vi "Run_Core.vi"(0 "Message Popup in":refnum<class "Wait.lvclass">, 11 "error in (no error)":errorcluster) -> (4 "Message Popup out":refnum<class "Wait.lvclass">, 6 "Return":variant, 15 "error out":errorcluster)   [LabVIEW 2016, in "Wait.lvclass"]
uses:
  Wait.lvclass
  Wait.lvclass/Wait.ctl
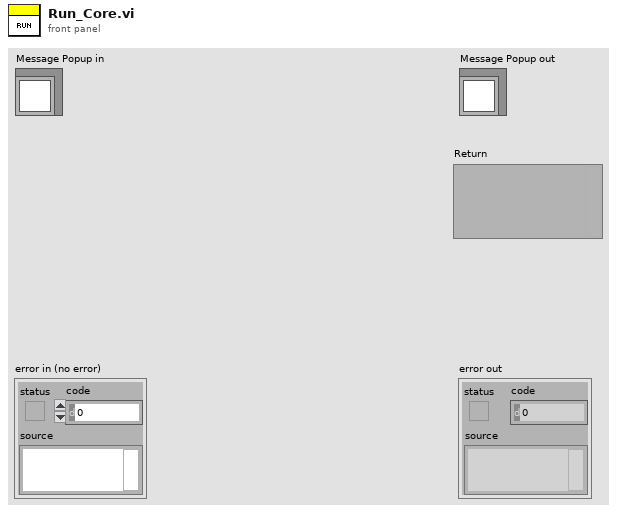
[diagram p1: front panel]
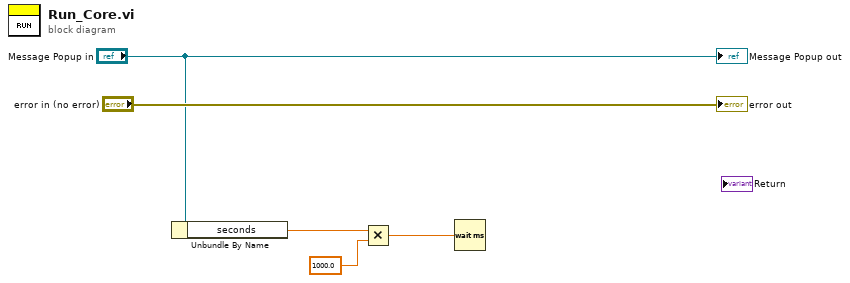
[diagram p0: block diagram]
diagram:
  n1 = Unbundle By Name("Message Popup in") -> ("seconds"=w3:dbl)
  n2 = Multiply(x=w3, y=1000.0) -> (x*y=w1:dbl)
  n3 = Wait (ms)(milliseconds to wait=w1) -> ()  [unwired: 1 out]
  "error out" <- "error in (no error)"
  "Message Popup out" <- "Message Popup in"
